vi "Write I16.vi"(8 "error in":errorcluster, 10 "element":T1, 11 "session in":u32) -> (0 "error out":errorcluster, 3 "session out":u32)   [LabVIEW 2018, in "Scalar IO Operations.lvlib"]
uses:
  Scalar IO Operations.lvlib
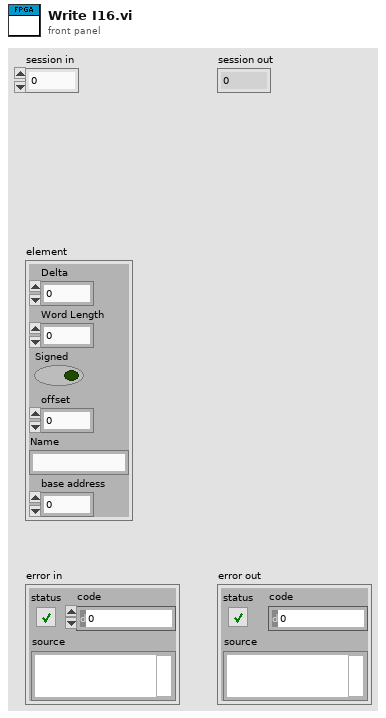
[diagram p1: front panel]
types:
  T1 = cluster{"Delta":dbl, "Word Length":i8, "Signed":bool, "offset":i32, "Name":string, "base address":i32}
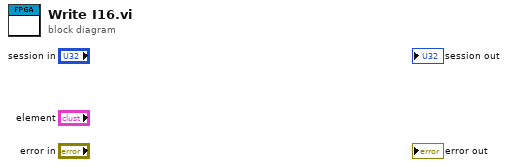
[diagram p0: block diagram]
diagram:
